vi "Drive_SetMotorsSpeed.vi"(8 "error in":errorcluster, 9 "Right_Speed":dbl min=-1.0 max=1.0, 10 "Left_Speed":dbl min=-1.0 max=1.0) -> (0 "error out":errorcluster)   [LabVIEW 2009, in "Drive.lvlib"]
uses:
  Drive.lvlib
  PWM/PWM_Name.ctl
  Motor.lvlib
  PWM.lvlib
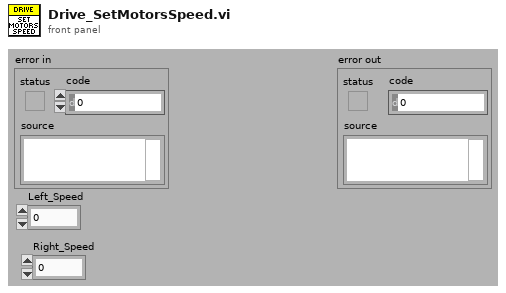
[diagram p1: front panel]
types:
  T1 = typedef "PWM.lvlib/PWM_Name.ctl" = u16
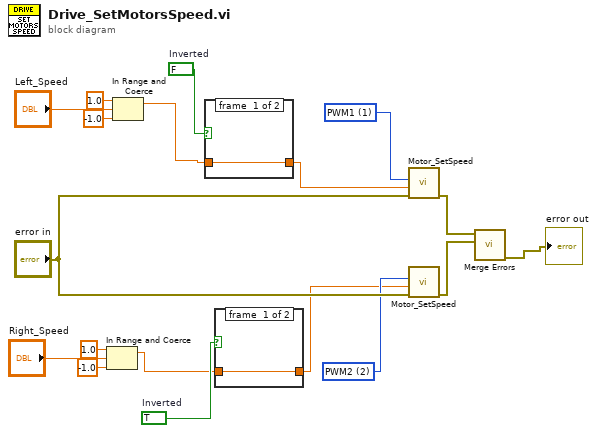
[diagram p0: block diagram]
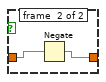
[diagram p2: hidden frame]
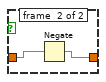
[diagram p3: hidden frame]
diagram:
  w3 = TRUE  # Inverted
  w4 = FALSE  # Inverted
  w7 = T1 2 items=["Invalid"=0, "PWM1"=1, "PWM2"=2, "PWM9"=9, "PWM10"=10] ("PWM_Channel")
  w8 = T1 1 items=["Invalid"=0, "PWM1"=1, "PWM2"=2, "PWM9"=9, "PWM10"=10] ("PWM_Channel")
  n1 = In Range and Coerce(upper limit=1.0, x="Right_Speed", lower limit=-1.0) -> (coerced(x)=w1:dbl)  [unwired: 1 out]
  n2 = In Range and Coerce(upper limit=1.0, x="Left_Speed", lower limit=-1.0) -> (coerced(x)=w6:dbl)  [unwired: 1 out]
  n3 = case shown="True" w4 {
    tunnel: w6 -> [w19 w20]
    tunnel: [w19 w21] -> w5
    frame #0 {
    }
    frame #1 {
      n4 = Negate(x=w20) -> (-x=w21:dbl)
    }
  }
  n5 = case shown="False" w3 {
    tunnel: w1 -> [w22 w23]
    tunnel: [w22 w24] -> w2
    frame #0 {
    }
    frame #1 {
      n6 = Negate(x=w23) -> (-x=w24:dbl)
    }
  }
  n7 = call "Motor_SetSpeed.vi"("error in"="error in", "Speed"=w5, "PWM_Channel"=w8) -> ("error out"=w17:errorcluster)  [unwired: 8 in]
  n8 = call "Motor_SetSpeed.vi"("error in"="error in", "Speed"=w2, "PWM_Channel"=w7) -> ("error out"=w16:errorcluster)  [unwired: 8 in]
  n9 = call <vilib>:"Merge Errors.vi"("error in 2 (no error)"=w16, "error in 1 (no error)"=w17) -> ("error out"=→"error out":errorcluster)  [unwired: 5 in]
